vi "setRunState.vi"(8 "error in (no error)":errorcluster, 10 "Runstate":T1, 11 "ScopeKeysight in":refnum<class "ScopeKeysight.lvclass">) -> (0 "error out":errorcluster, 3 "ScopeKeysight out":refnum<class "ScopeKeysight.lvclass">)   [LabVIEW 2023, in "ScopeKeysight.lvclass"]
doc: "<b>Author:</b> Wolfgang\n<b>Description:</b> Set Scope Runstate."
uses:
  ScopeKeysight.lvclass
  Data/scopeRunState.ctl
  ScopeKeysight.lvclass/ScopeKeysight.ctl
  Driver/Keysight-DSQx3014T.lvlib
  sweScope.lvlib
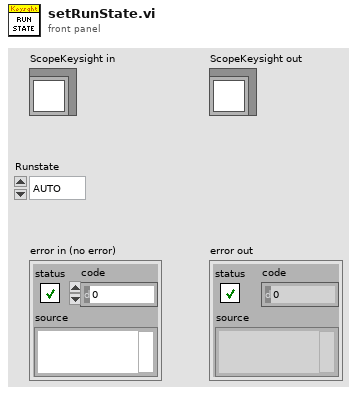
[diagram p1: front panel]
types:
  T1 = typedef "sweScope.lvlib/scopeRunState.ctl" = enum16{"AUTO", "NORMAL", "SINGLE"}
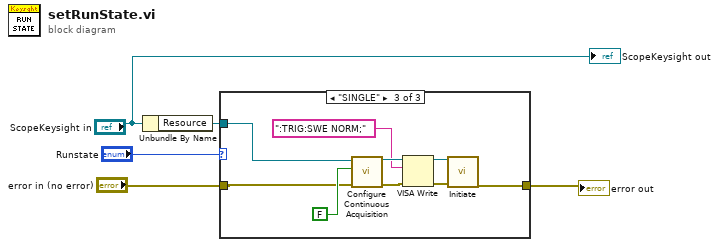
[diagram p0: block diagram]
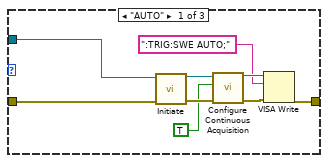
[diagram p2: hidden frame]
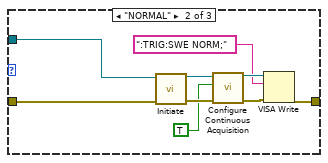
[diagram p3: hidden frame]
diagram:
  n1 = Unbundle By Name("ScopeKeysight in") -> ("Resource"=w4:refnum<visa-resource-name>)
  n2 = case shown="\"SINGLE\"" "Runstate" {
    tunnel: w4 -> [w14 w23 w25]
    tunnel: [w7 w16 w26] -> w2
    tunnel: "error in (no error)" -> [w11 w20 w24]
    frame "AUTO" {
      n3 = call "Initiate.vi"("error in (no error)"=w11, "VISA resource name"=w14) -> ("error out"=w12:errorcluster, "VISA resource name out"=w13:refnum<visa-resource-name>)  [unwired: 8 in]
      n4 = call "Configure Continuous Acquisition.vi"("error in (no error)"=w12, "Enable Continuous Acquisition Mode (T:Enable)"=TRUE, "VISA resource name"=w13) -> ("error out"=w8:errorcluster, "VISA resource name out"=w9:refnum<visa-resource-name>)  [unwired: 7 in]
      n5 = VISA Write(VISA resource name=w9, write buffer=":TRIG:SWE AUTO;", error in (no error)=w8) -> (error out=w7:errorcluster)  [unwired: 2 out]
    }
    frame "NORMAL" {
      n6 = call "Initiate.vi"("error in (no error)"=w20, "VISA resource name"=w23) -> ("error out"=w21:errorcluster, "VISA resource name out"=w22:refnum<visa-resource-name>)  [unwired: 8 in]
      n7 = call "Configure Continuous Acquisition.vi"("error in (no error)"=w21, "Enable Continuous Acquisition Mode (T:Enable)"=TRUE, "VISA resource name"=w22) -> ("error out"=w17:errorcluster, "VISA resource name out"=w18:refnum<visa-resource-name>)  [unwired: 7 in]
      n8 = VISA Write(VISA resource name=w18, write buffer=":TRIG:SWE NORM;", error in (no error)=w17) -> (error out=w16:errorcluster)  [unwired: 2 out]
    }
    frame "SINGLE" {
      n9 = call "Configure Continuous Acquisition.vi"("error in (no error)"=w24, "Enable Continuous Acquisition Mode (T:Enable)"=FALSE, "VISA resource name"=w25) -> ("error out"=w30:errorcluster, "VISA resource name out"=w31:refnum<visa-resource-name>)  [unwired: 7 in]
      n10 = VISA Write(VISA resource name=w31, write buffer=":TRIG:SWE NORM;", error in (no error)=w30) -> (VISA resource name out=w28:refnum<visa-resource-name>, error out=w27:errorcluster)  [unwired: 1 out]
      n11 = call "Initiate.vi"("error in (no error)"=w27, "VISA resource name"=w28) -> ("error out"=w26:errorcluster)  [unwired: 8 in, 1 out]
    }
  }
  "error out" <- w2
  "ScopeKeysight out" <- "ScopeKeysight in"
